vi "xlsxDriver.vi"(8 "error in":errorcluster, 11 "XML File Path":path=path "C:/LabviewFiles/LabView/learning(Lee)/LVU examples/xmlParsing/ETNT22116.xml") -> (0 "error out":errorcluster)   [LabVIEW 2018]
uses:
  Global Variables.vi
panel:
  out "outputFeature":string[](array[string])
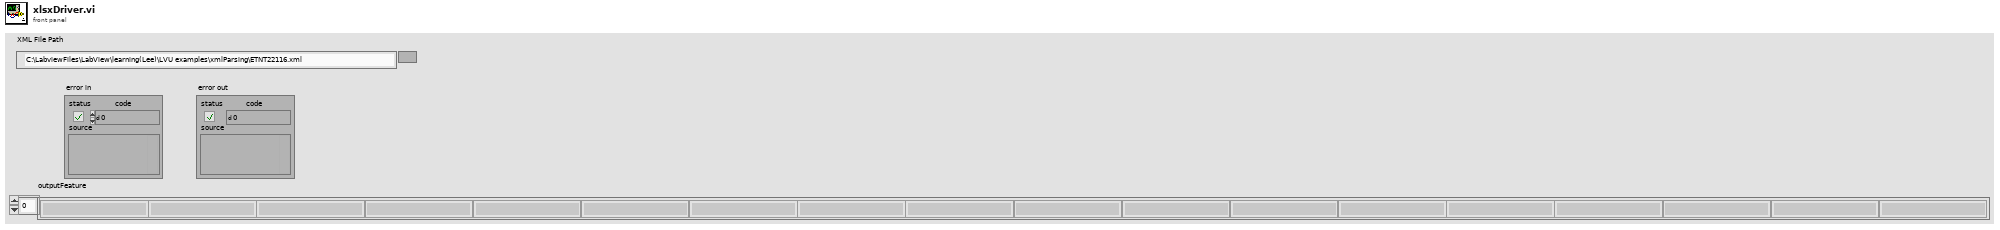
[diagram p1: front panel]
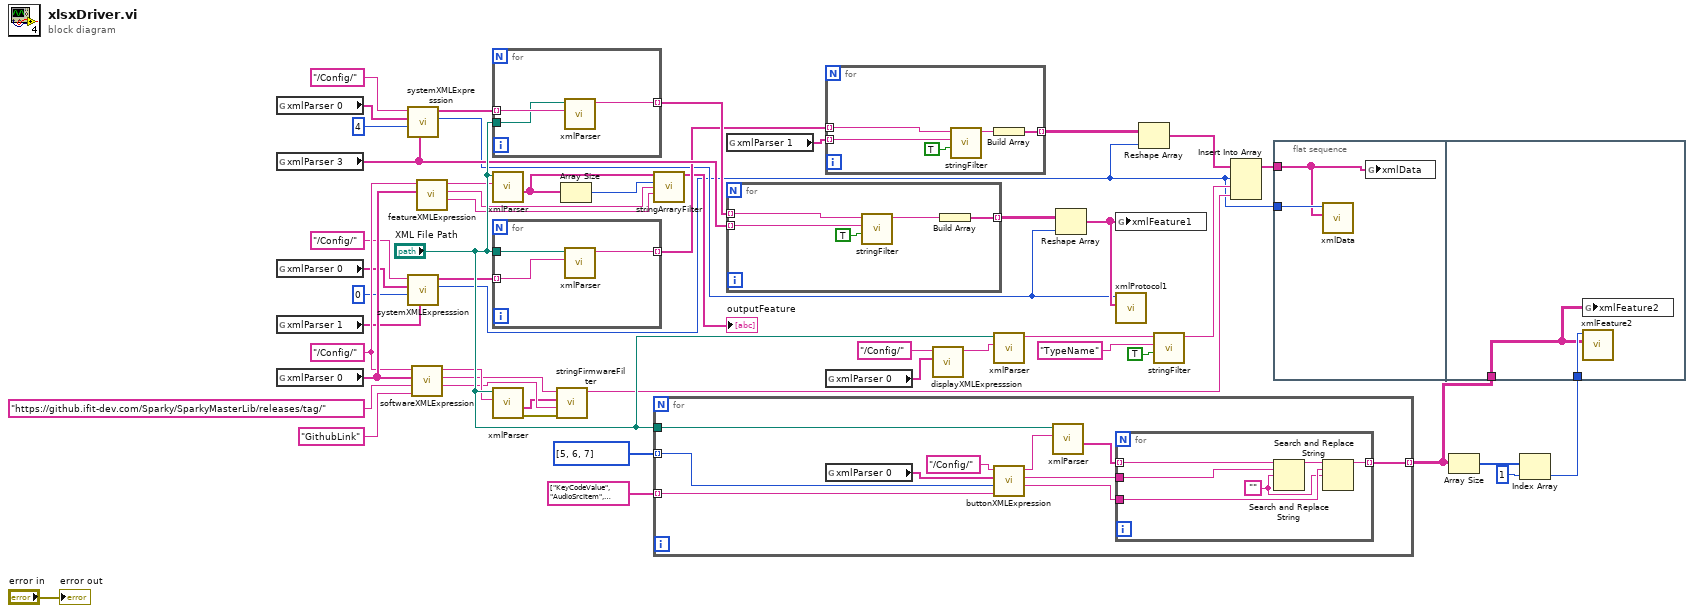
[diagram p0: block diagram]
diagram:
  w36 = "/Config/" ("String in")
  n1 = global read "Global Variables.vi" "xmlParser 0"() -> (w42:string[])
  n2 = global read "Global Variables.vi" "xmlParser 3"() -> (w39:string[])
  n3 = global read "Global Variables.vi" "xmlParser 0"() -> (w13:string[])
  n4 = global read "Global Variables.vi" "xmlParser 1"() -> (w11:string[])
  n5 = global read "Global Variables.vi" "xmlParser 0"() -> (w37:string[])
  n6 = call "systemXMLExpresssion.vi"("xmlParser 1"=w39, "index"=4, "xmlParser 0"=w42, "String"="/Config/") -> ("Numeric"=w8:i32, "output array"=w41:string[])  [unwired: 6 in]
  n7 = call "systemXMLExpresssion.vi"("xmlParser 1"=w11, "index"=0, "xmlParser 0"=w13, "String"="/Config/") -> ("Numeric"=w3:i32, "output array"=w12:string[])  [unwired: 6 in]
  n8 = call "softwareXMLExpression.vi"("postValue"="GithubLink", "preValue"="https://github.ifit-dev.com/Sparky/SparkyMasterLib/releases/tag/", "xmlParser 0"=w37, "String in"=w36) -> ("filter2"=w27:string, "filter1"=w28:string, "swXMLExpression"=w29:string)  [unwired: 5 in]
  n9 = call "featureXMLExpression.vi"("xmlParser 0"=w37, "String in"=w36) -> ("string"=w32:string, "String 2"=w31:string, "String"=w33:string)  [unwired: 7 in]
  n10 = for {
    tunnel: w41 -> [w53] mode=indexing
    tunnel: [w54] -> w40 mode=indexing
    tunnel: "XML File Path" -> [w52]
    n11 = call "xmlParser.vi"("XPath Expression"=w53, "XML File Path"=w52) -> ("outputString"=w54:string)  [unwired: 6 in, 3 out]
  }
  n12 = call "xmlParser.vi"("XPath Expression"=w33, "XML File Path"="XML File Path") -> ("outputArray"=w34:string[])  [unwired: 6 in, 3 out]
  n13 = for {
    tunnel: "XML File Path" -> [w56]
    tunnel: w12 -> [w55] mode=indexing
    tunnel: [w57] -> w17 mode=indexing
    n14 = call "xmlParser.vi"("XPath Expression"=w55, "XML File Path"=w56) -> ("outputString"=w57:string)  [unwired: 6 in, 3 out]
  }
  n15 = call "xmlParser.vi"("XPath Expression"=w29, "XML File Path"="XML File Path") -> ("error out"=w7:errorcluster, "outputArray"=w6:string[])  [unwired: 6 in, 2 out]
  n16 = call "stringFirmwareFilter.vi"("error in (no error)"=w7, "filter2"=w27, "inputArray"=w6, "filter1"=w28) -> ("result string"=w30:string)  [unwired: 7 in]
  n17 = Array Size(array=w34) -> (size(s)=w35:i32)
  n18 = call "stringArraryFilter.vi"("inputFeature"=w34, "stringLength"=w35, "stringFilterBegin"=w31, "stringFilterEnd"=w32) -> ("outputFeature"=→"outputFeature":string[])  [unwired: 11 in]
  n19 = for {
    tunnel: string[] ["KeyCodeValue", "AudioSrcItem", "PulseDriverItem"] -> [w61] mode=indexing
    tunnel: i32[] [5, 6, 7] -> [w60] mode=indexing
    tunnel: [w59] -> w1 mode=indexing
    tunnel: "XML File Path" -> [w58]
    n20 = global read "Global Variables.vi" "xmlParser 0"() -> (w67:string[])
    n21 = call "buttonXMLExpression.vi"("preValue"=w61, "index"=w60, "xmlParser 0"=w67, "String 4"="/Config/" ("String")) -> ("stringFilter2"=w64:string, "stringFilter1"=w62:string, "buttonXMLExpression"=w65:string)  [unwired: 5 in]
    n22 = call "xmlParser.vi"("XPath Expression"=w65, "XML File Path"=w58) -> ("outputArray"=w63:string[])  [unwired: 6 in, 3 out]
    n23 = for {
      tunnel: w62 -> [w73]
      tunnel: w64 -> [w71]
      tunnel: w63 -> [w69] mode=indexing
      tunnel: [w68] -> w59 mode=indexing
      w70 = ""
      n24 = Search and Replace String(input string=w69, search string=w73, replace string=w70) -> (result string=w72:string)  [unwired: 5 in, 3 out]
      n25 = Search and Replace String(input string=w72, search string=w71, replace string=w70) -> (result string=w68:string)  [unwired: 5 in, 3 out]
    }
  }
  n26 = global read "Global Variables.vi" "xmlParser 1"() -> (w16:string[])
  n27 = for {
    tunnel: [w78] -> w38 mode=indexing
    tunnel: w40 -> [w75] mode=indexing
    tunnel: w39 -> [w74] mode=indexing
    n28 = call "stringFilter.vi"("Active"=TRUE, "filterString"=w74, "inputString"=w75) -> ("resultString"=w77:string)  [unwired: 7 in, 1 out]
    n29 = Build Array(w77) -> (w78:string[])
  }
  n30 = for {
    tunnel: w16 -> [w81] mode=indexing
    tunnel: w17 -> [w82] mode=indexing
    tunnel: [w83] -> w18 mode=indexing
    n31 = call "stringFilter.vi"("Active"=TRUE, "filterString"=w81, "inputString"=w82) -> ("resultString"=w80:string)  [unwired: 7 in, 1 out]
    n32 = Build Array(w80) -> (w83:string[])
  }
  n33 = global read "Global Variables.vi" "xmlParser 0"() -> (w20:string[])
  n34 = call "displayXMLExpresssion.vi"("xmlParser 0"=w20, "String in"="/Config/") -> ("String out"=w21:string)  [unwired: 9 in]
  n35 = call "xmlParser.vi"("XPath Expression"=w21, "XML File Path"="XML File Path") -> ("outputString"=w22:string)  [unwired: 6 in, 3 out]
  n36 = Reshape Array(w38, w8) -> (w9:string[])
  n37 = global write "Global Variables.vi" "xmlFeature1"(w9) -> ()
  n38 = call "xmlProtocol1.vi"("Array"=w9, "Numeric"=w8) -> ()  [unwired: 10 in]
  n39 = Reshape Array(w18, w3) -> (w25:string[])
  n40 = call "stringFilter.vi"("Active"=TRUE, "filterString"="TypeName", "inputString"=w22) -> ("resultString"=w26:string)  [unwired: 7 in, 1 out]
  n41 = Insert Into Array(array=w25, index=w3, new element #1=w26, new element #2=w30) -> (w4:string[])
  n42 = flat-sequence {
    tunnel: w4 -> [w84]
    tunnel: w3 -> [w85]
    tunnel: w2 -> [w87]
    tunnel: w1 -> [w86]
    frame #0 {
      n43 = call "xmlData.vi"("Array"=w84, "Numeric"=w85) -> ()  [unwired: 10 in]
      n44 = global write "Global Variables.vi" "xmlData"(w84) -> ()
    }
    frame #1 {
      n45 = global write "Global Variables.vi" "xmlFeature2"(w86) -> ()
      n46 = call "xmlFeature2.vi"("Array"=w86, "Numeric"=w87) -> ()  [unwired: 10 in]
    }
  }
  n47 = Array Size(array=w1) -> (size(s)=w49:i32[])
  n48 = Index Array(array=w49, index=1) -> (element=w2:i32)
  "error out" <- "error in"
